vi "Deploy_SetImage.vi"(8 "error in (no error)":errorcluster, 9 "DevInfo":T3={"Hostname"="", "IPAddress"="", "MAC"="", "SerialNum"="", "Model"="", "Status"="", "FW"="", "OSDesc"="", "ImgTitle"="", "ImgDesc"="", "ImgVer"="", "ImgID"="", "IP Address Request Mode"=1, "SubnetMask"="", "Gateway"="", "DNSServer"=""} {"IP Address Request Mode" items=["Static"=1, "DHCP/Link-Local"=2, "Link-Local Only"=4, "DHCP Only"=8]}, 10 "AppImage Properties":T1, 11 "Selected Image File":path) -> (0 "error out":errorcluster)   [LabVIEW 2021]
uses:
  TypeDefs/DevInfo.ctl
  TypeDefs/AppImageProperties.ctl
  TypeDefs/FPGA_Properties_Element.ctl
  TypeDefs/TargetAccess.ctl
  <vilib>/nisyscfg/Network Settings Image.ctl
  <vilib>/nisyscfg/Set System Image (File).vi
  <vilib>/nisyscfg/Close (System).vi
  <vilib>/nisyscfg/nisyscfg.lvlib
panel:
  in  "Stop Checking for Events":bool
  out "Progress":i8(slide) scale=0.0..100.0
  out "Status":string
  # "Deploying Image"
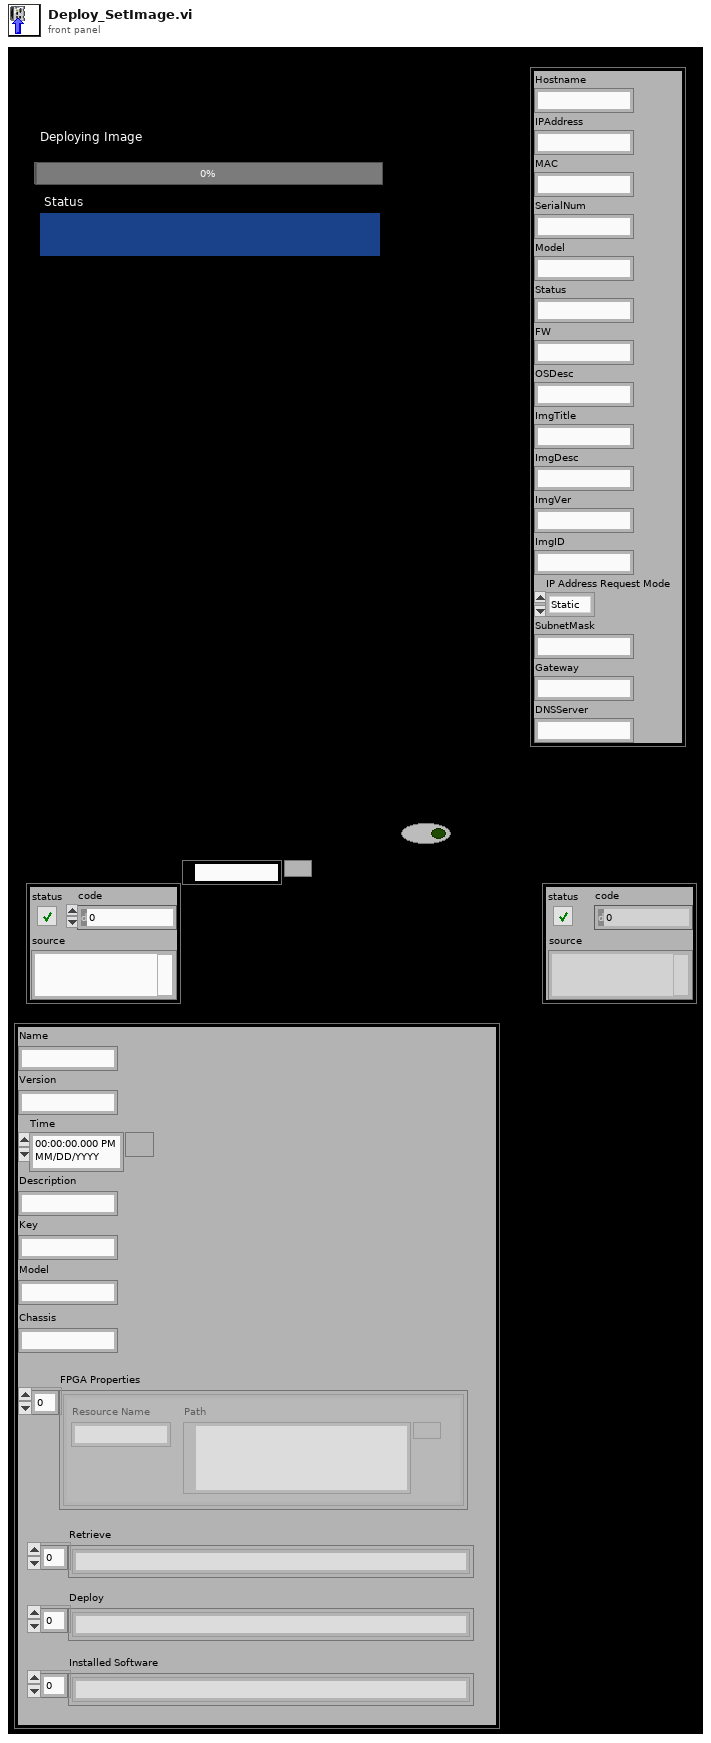
[diagram p1: front panel]
types:
  T1 = typedef "AppImageProperties.ctl" = cluster{"Name":string, "Version":string, "Time":timestamp, "Description":string, "Key":string, "Chassis":string, "FPGA Properties":T2[], "Model":string, "Retrieve":string[], "Deploy":string[], "Installed Software":string[]}
  T2 = typedef "FPGA_Properties_Element.ctl" = cluster{"Resource Name":string, "Path":path}
  T3 = typedef "DevInfo.ctl" = cluster{"Hostname":string, "IPAddress":string, "MAC":string, "SerialNum":string, "Model":string, "Status":string, "FW":string, "OSDesc":string, "ImgTitle":string, "ImgDesc":string, "ImgVer":string, "ImgID":string, "IP Address Request Mode":i32, "SubnetMask":string, "Gateway":string, "DNSServer":string}
  T4 = typedef "TargetAccess.ctl" = enum16{"Read-Only", "Admin"}
  T5 = typedef "nisyscfg.lvlib/Network Settings Image.ctl" = u32
  T6 = enum32{"state changed", "beginning restart", "getting file", "putting file", "creating directory", "deleting file", "deleting directory", "enumerating file system", "renaming file", "current component", "operation progress", "downloading file", "unpacking file", "running install script", "creating image", "validating image", "applying image", "beginning format", "completing format"}
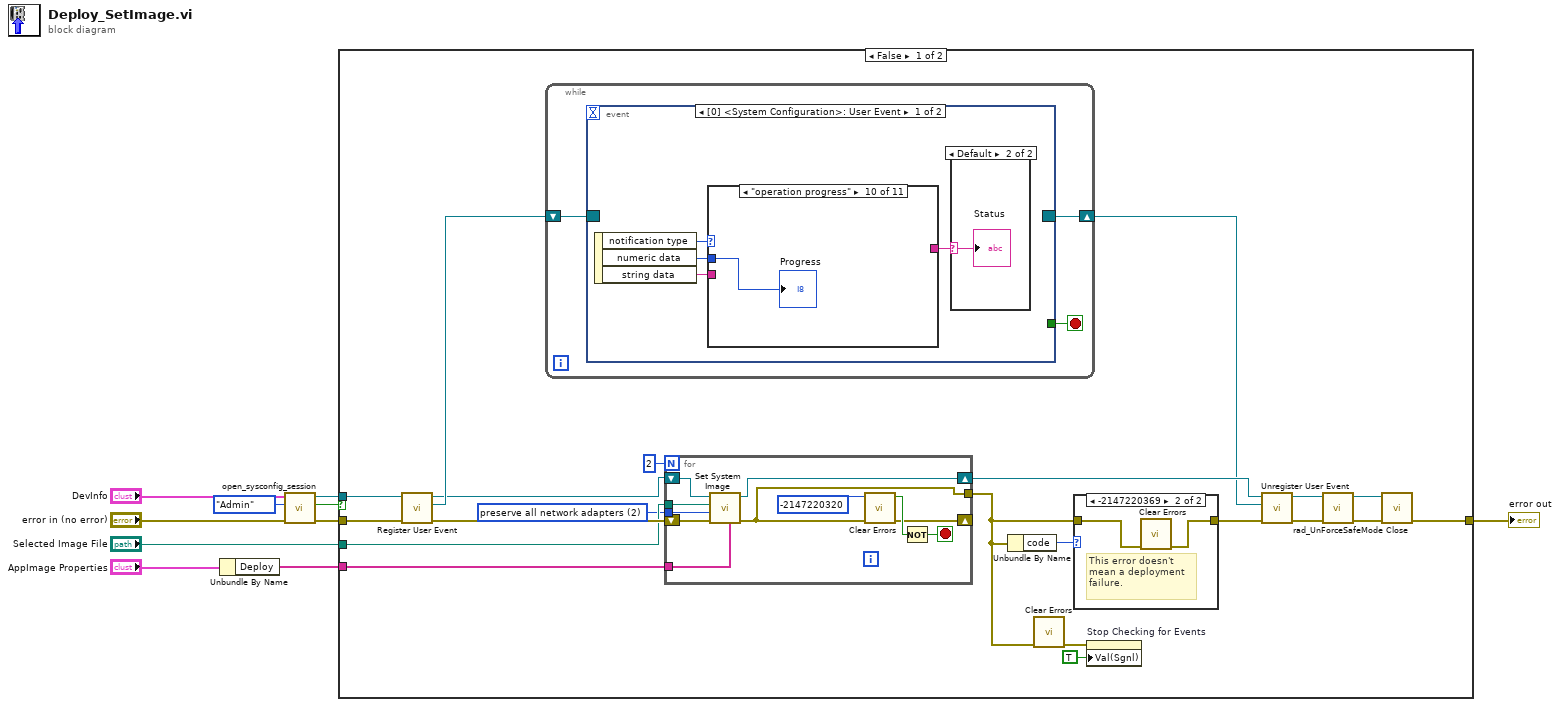
[diagram p0: block diagram]
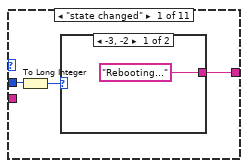
[diagram p4: hidden frame]
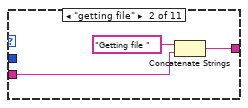
[diagram p6: hidden frame]
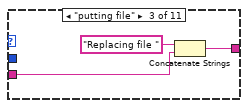
[diagram p7: hidden frame]
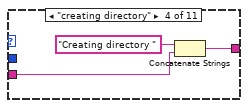
[diagram p8: hidden frame]
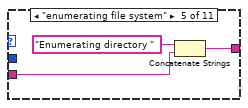
[diagram p9: hidden frame]
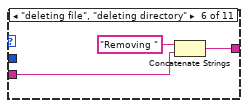
[diagram p10: hidden frame]
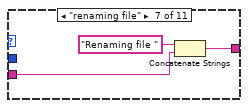
[diagram p11: hidden frame]
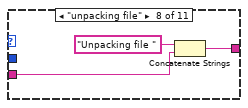
[diagram p12: hidden frame]
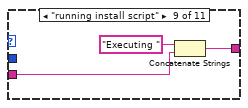
[diagram p13: hidden frame]
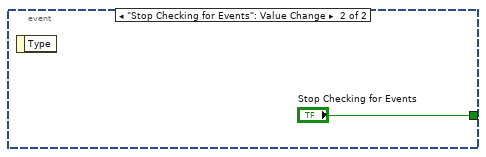
[diagram p15: hidden frame]
diagram:
  n1 = Unbundle By Name("AppImage Properties") -> ("Deploy"=w2:string[])
  n2 = call "open_sysconfig_session.vi"("error in (no error)"="error in (no error)", "Target Access"=TargetAccess."Admin", "DevInfo"="DevInfo") -> ("error out"=w6:errorcluster, "Cancelled"=w7:bool, "Session Out"=w5:refnum<k21>)  [unwired: 6 in]
  n3 = case shown="False" w7 {
    tunnel: w6 -> [w29 w84]
    tunnel: w5 -> [w30 _]
    tunnel: "Selected Image File" -> [w25 _]
    tunnel: w2 -> [w23 _]
    tunnel: [w12 w84] -> w1
    frame False {
      w24 = T5 2 items=["reset all network adapters", "preserve primary, reset others", "preserve all network adapters", "preserve primary, apply others", "apply primary, reset others", "apply primary, preserve others", "apply all network adapters"] ("network settings (apply all adapters)")
      n4 = call <vilib>:"Register User Event.vi"("error in (no error)"=w29, "Session in"=w30) -> ("error out"=w26:errorcluster, "Event Registration out"=w31:refnum<event-registration>, "Session out"=w27:refnum<k21>)  [unwired: 7 in]
      n5 = while {
        shift-right: [w46] -> w17
        shift-left: w31 -> [w48]
        stop <- w47 stop-if-true
        n6 = event shown="[0] <System Configuration>: User Event" {
          selector: w48 -> [_ _]
          dyn-events: [_ _] -> w46
          timeout: _ -> [_ _]
          tunnel: [_ "Stop Checking for Events"] -> w47
          event User Event {
            n7 = event-data() -> ("notification type"=w52:T6, "numeric data"=w50:u32, "string data"=w51:string)  [unwired: 1 in]
            n8 = case shown="\"operation progress\"" w52 {
              tunnel: [w54 w58 w61 w64 w67 w70 w73 w76 w79 _ _] -> w49
              tunnel: w51 -> [_ w59 w62 w65 w68 w71 w74 w77 w80 _ _]
              tunnel: w50 -> [w56 _ _ _ _ _ _ _ _ w82 _]
              frame "state changed" {
                n9 = To Long Integer(number=w56) -> (32bit integer=w55:i32)
                n10 = case shown="-3, -2" w55 {
                  tunnel: ["Rebooting..." _] -> w54
                  frame -3, -2 {
                  }
                  frame Default {
                  }
                }
              }
              frame "getting file" {
                n11 = Concatenate Strings("Getting file " ("Status"), w59) -> (w58:string)
              }
              frame "putting file" {
                n12 = Concatenate Strings("Replacing file " ("Status"), w62) -> (w61:string)
              }
              frame "creating directory" {
                n13 = Concatenate Strings("Creating directory " ("Status"), w65) -> (w64:string)
              }
              frame "enumerating file system" {
                n14 = Concatenate Strings("Enumerating directory " ("Status"), w68) -> (w67:string)
              }
              frame "deleting file", "deleting directory" {
                n15 = Concatenate Strings("Removing " ("Status"), w71) -> (w70:string)
              }
              frame "renaming file" {
                n16 = Concatenate Strings("Renaming file " ("Status"), w74) -> (w73:string)
              }
              frame "unpacking file" {
                n17 = Concatenate Strings("Unpacking file " ("Status"), w77) -> (w76:string)
              }
              frame "running install script" {
                n18 = Concatenate Strings("Executing " ("Status"), w80) -> (w79:string)
              }
              frame "operation progress" {
                "Progress" <- w82
              }
              frame Default {
              }
            }
            n19 = case shown="Default" w49 {
              selector: w49 -> [_ w53]
              frame "" {
              }
              frame Default {
                "Status" <- w53
              }
            }
          }
          event "Stop Checking for Events": Value Change {
            n20 = event-data() -> ()  [unwired: 1 in, 1 out]
          }
        }
      }
      n21 = for {
        N: 2 -> [_]
        tunnel: w25 -> [w45]
        tunnel: w24 -> [w43]
        tunnel: w23 -> [w41]
        tunnel: [w36] -> w21
        shift-right: [w38] -> _
        shift-left: w26 -> [w42]
        shift-right: [w37] -> w18
        shift-left: w27 -> [w44]
        stop <- w40 stop-if-true
        n22 = call-poly <vilib>:"Set System Image.vi"("File and Directory Blacklist"=w41, "error in (no error)"=w42, "Network Settings (preserve primary adapter, apply others)"=w43, "Source File"=w45, "Session in"=w44) -> ("error out"=w36:errorcluster, "Session out"=w37:refnum<k21>)  [unwired: 5 in]
        n23 = call <vilib>:"Clear Errors.vi"("error in (no error)"=w36, "specific error code to clear (0: all)"=-2147220320) -> ("error out"=w38:errorcluster, "specific error cleared?"=w39:bool)  [unwired: 4 in]
        n24 = Not(x=w39) -> (.not. x?=w40:bool)
      }
      n25 = Unbundle By Name(w21) -> ("code"=w22:i32)
      n26 = call <vilib>:"Clear Errors.vi"("error in (no error)"=w21) -> ("error out"=w20:errorcluster)  [unwired: 5 in, 1 out]
      n27 = case shown="-2147220369" w22 {
        tunnel: w21 -> [w32 w34]
        tunnel: [w32 w33] -> w19
        frame Default {
        }
        frame -2147220369 {
          # "This error doesn't\nmean a deployment\nfailure."
          n28 = call <vilib>:"Clear Errors.vi"("error in (no error)"=w34) -> ("error out"=w33:errorcluster)  [unwired: 5 in, 1 out]
        }
      }
      n29 = property on="Stop Checking for Events" class="Bool (strict)"(error in=w20, "Val(Sgnl)"=TRUE ("Value (Signaling)")) -> ()  [unwired: 1 in, 2 out]
      n30 = call <vilib>:"Unregister User Event.vi"("error in (no error)"=w19, "Event Registration in"=w17, "Session in"=w18) -> ("error out"=w15:errorcluster, "Session out"=w16:refnum<k21>)  [unwired: 7 in]
      n31 = call "rad_UnForceSafeMode.vi"("error in (no error)"=w15, "Target in"=w16) -> ("error out"=w13:errorcluster, "Target out"=w14:refnum<k21>)  [unwired: 8 in]
      n32 = call-poly <vilib>:"Close.vi"("error in (no error)"=w13, "Session in"=w14) -> ("error out"=w12:errorcluster)  [unwired: 9 in]
    }
    frame True {
    }
  }
  "error out" <- w1
